vi "Handle Request.vi"(7 "Processing In":refnum<class "Processing.lvclass">, 11 "PathValidation in":refnum<class "PathValidation.lvclass">) -> (0 "error out":errorcluster, 5 "Processing":refnum<class "Processing.lvclass">)   [LabVIEW 2023, in "HTTP Server.lvlib" / "PathValidation.lvclass"]
uses:
  PathValidation.lvclass
  Processing/Processing.lvclass
  Processing/Processing.lvclass/Processing.ctl
  lv-http-util/HTTP Utils/Request/Request.lvclass/Request.ctl
  lv-uri/URI/URI/URI.lvclass/URI.ctl
  lv-http-util/HTTP Utils/Request/Get Target URI.vi
  lv-uri/URI/URI/Path String.vi
  <vilib>/Utility/error.llb/Error Cluster From Error Code.vi
  <vilib>/regexp/Match Regular Expression.xnode
  <vilib>/ErrorRing/Error Ring.xnode
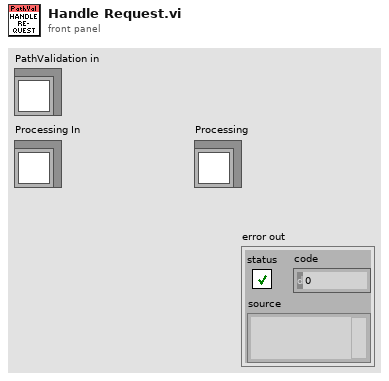
[diagram p1: front panel]
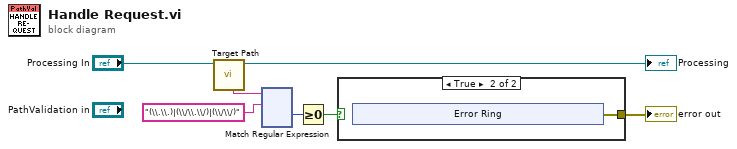
[diagram p0: block diagram]
diagram:
  n1 = call "Target Path.vi"("Processing in"="Processing In") -> ("Processing out"=→"Processing":refnum<class "Processing.lvclass">, "Target Path"=w3:string)  [unwired: 9 in]
  n2 = xnode "Match Regular Expression"("input string"=w3, "regular expression"="(\\.\\.)|(\\/\\.\\/)|(\\/\\/)") -> ("offset past match"=w6:i32)  [unwired: 4 in, 4 out]
  n3 = Greater Or Equal To 0?(x=w6) -> (x >= 0?=w5:bool)
  n4 = case shown="True" w5 {
    tunnel: [_ w8] -> w4
    frame False {
    }
    frame True {
      n5 = xnode "Error Ring"() -> ("error out"=w8:errorcluster)
    }
  }
  "error out" <- w4
